vi "Update State Value.vi"(8 "error in (no error)":errorcluster, 9 "New Value":i32, 10 "State":string, 11 "Channel Ref in":T1 format="%.0x") -> (0 "error out":errorcluster, 3 "Channel Ref out":T1=18446744073709551615 format="%.0x")   [LabVIEW 2017, in "SLSC Switch Scripting.lvlib"]
uses:
  SLSC Switch Scripting.lvlib
  <vilib>/NI Veristand/Custom Device API/Custom Device Item Ref.ctl
  <vilib>/NI VeriStand/Custom Device API/Custom Device API.lvlib
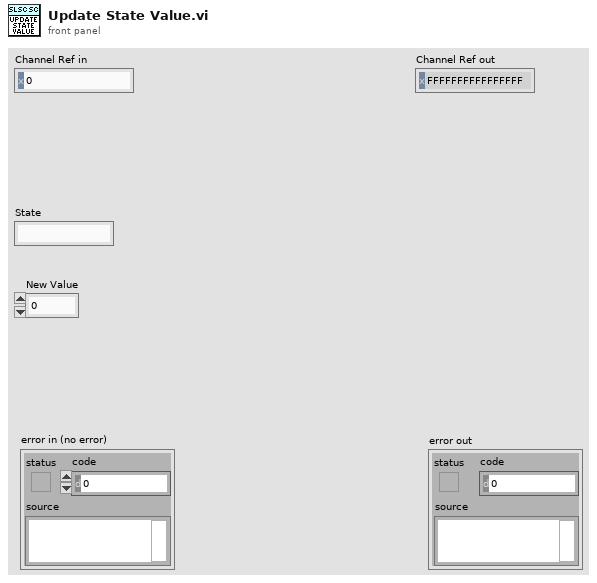
[diagram p1: front panel]
types:
  T1 = typedef "Custom Device API.lvlib/Custom Device Item Ref.ctl" = u64
  T2 = typedef "SLSC Switch Scripting.lvlib/Routing State.ctl" = cluster{"name":string, "description":string, "value":i32, "connection list":T3[]}
  T3 = typedef "SLSC Switch Scripting.lvlib/Connection.ctl" = cluster{"source":string, "destination":string}
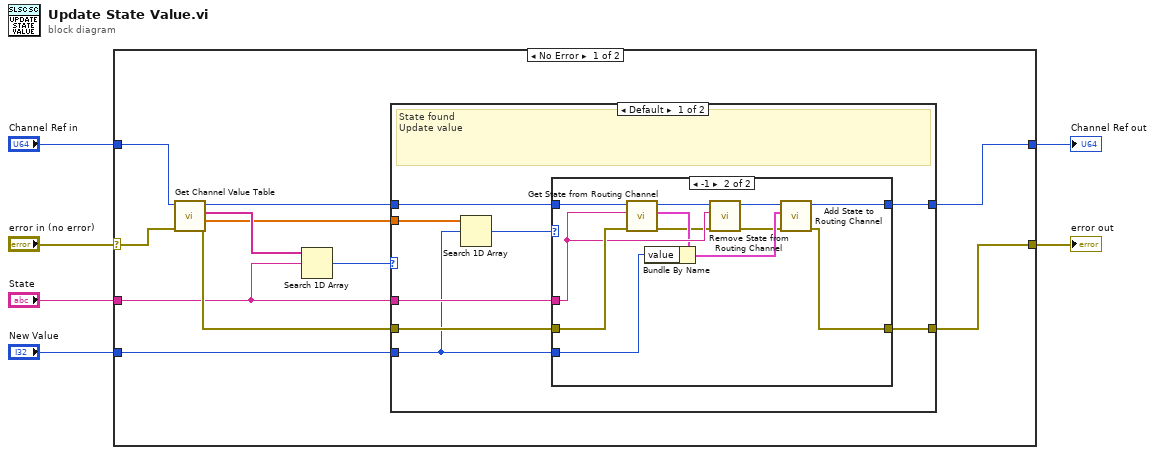
[diagram p0: block diagram]
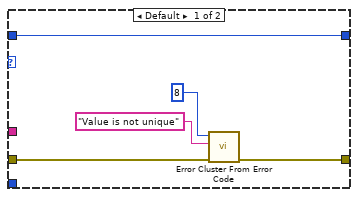
[diagram p2: hidden frame]
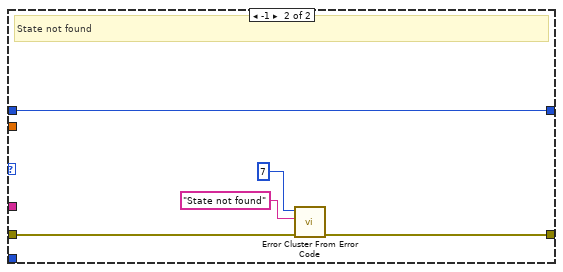
[diagram p3: hidden frame]
diagram:
  n1 = case shown="No Error" "error in (no error)" {
    selector: "error in (no error)" -> [w17 w49]
    tunnel: [w13 w49] -> w1
    tunnel: [w14 w48] -> w2
    tunnel: "State" -> [w11 _]
    tunnel: "New Value" -> [w8 _]
    tunnel: "Channel Ref in" -> [w7 w48]
    frame No Error {
      n2 = call "Get Channel Value Table.vi"("error in (no error)"=w17, "Channel Ref in"=w7) -> ("error out"=w15:errorcluster, "Values"=w10:dbl[], "States"=w12:string[], "Channel Ref out"=w16:T1)  [unwired: 6 in]
      n3 = Search 1D Array(1D array=w12, element=w11) -> (index of element=w9:i32)  [unwired: 1 in]
      n4 = case shown="Default" w9 {
        tunnel: w16 -> [w25 w43]
        tunnel: w15 -> [w24 w45]
        tunnel: w10 -> [w19 _]
        tunnel: [w20 w43] -> w14
        tunnel: [w22 w44] -> w13
        tunnel: w11 -> [w23 _]
        tunnel: w8 -> [w18 _]
        frame Default {
          # "State found\nUpdate value"
          n5 = Search 1D Array(1D array=w19, element=w18) -> (index of element=w21:i32)  [unwired: 1 in]
          n6 = case shown="-1" w21 {
            tunnel: w25 -> [w26 w42]
            tunnel: w24 -> [w28 w41]
            tunnel: w23 -> [_ w40]
            tunnel: [w27 w31] -> w22
            tunnel: [w26 w32] -> w20
            tunnel: w18 -> [_ w37]
            frame Default {
              n7 = call <vilib>:"Error Cluster From Error Code.vi"("error in (no error)"=w28, "error message (\"\")"="Value is not unique" ("error message (\"\")"), "error code (0)"=8) -> ("error out"=w27:errorcluster)  [unwired: 6 in]
            }
            frame -1 {
              n8 = call "Get State from Routing Channel.vi"("error in (no error)"=w41, "State"=w40, "Channel Ref in"=w42) -> ("error out"=w36:errorcluster, "Routing State"=w39:T2, "Channel Ref out"=w35:T1)  [unwired: 6 in]
              n9 = Bundle By Name(cluster=w39, "value"=w37) -> (w38:T2)
              n10 = call "Remove State from Routing Channel.vi"("error in (no error)"=w36, "State"=w40, "Channel Ref in"=w35) -> ("error out"=w33:errorcluster, "Channel Ref out"=w34:T1)  [unwired: 7 in]
              n11 = call "Add State to Routing Channel.vi"("error in (no error)"=w33, "Routing State"=w38, "Channel Ref in"=w34) -> ("error out"=w31:errorcluster, "Channel Ref out"=w32:T1)  [unwired: 7 in]
            }
          }
        }
        frame -1 {
          # "State not found"
          n12 = call <vilib>:"Error Cluster From Error Code.vi"("error in (no error)"=w45, "error message (\"\")"="State not found" ("error message (\"\")"), "error code (0)"=7) -> ("error out"=w44:errorcluster)  [unwired: 6 in]
        }
      }
    }
    frame Error {
    }
  }
  "Channel Ref out" <- w2
  "error out" <- w1
